vi "Wait for Stop Notification.vi"(8 "error in (no error)":errorcluster, 9 "Loop Period [ms]":i32, 11 "Event Registration Refnum in":refnum<event-registration>) -> (0 "error out":errorcluster, 1 "Stop Received?":bool, 3 "Event Registration Refnum out":refnum<event-registration>)   [LabVIEW 2020, in "Helper Loop.lvclass"]
uses:
  Helper Loop.lvclass
  Process/Protected/Broadcasting/Broadcast Message Cluster.ctl
  Broadcast Event Helpers/Broadcast Event Helpers.lvlib
  Process/Process.lvclass
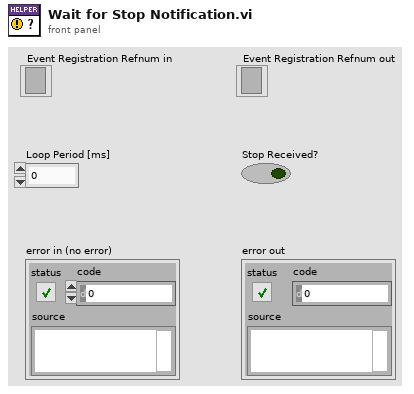
[diagram p1: front panel]
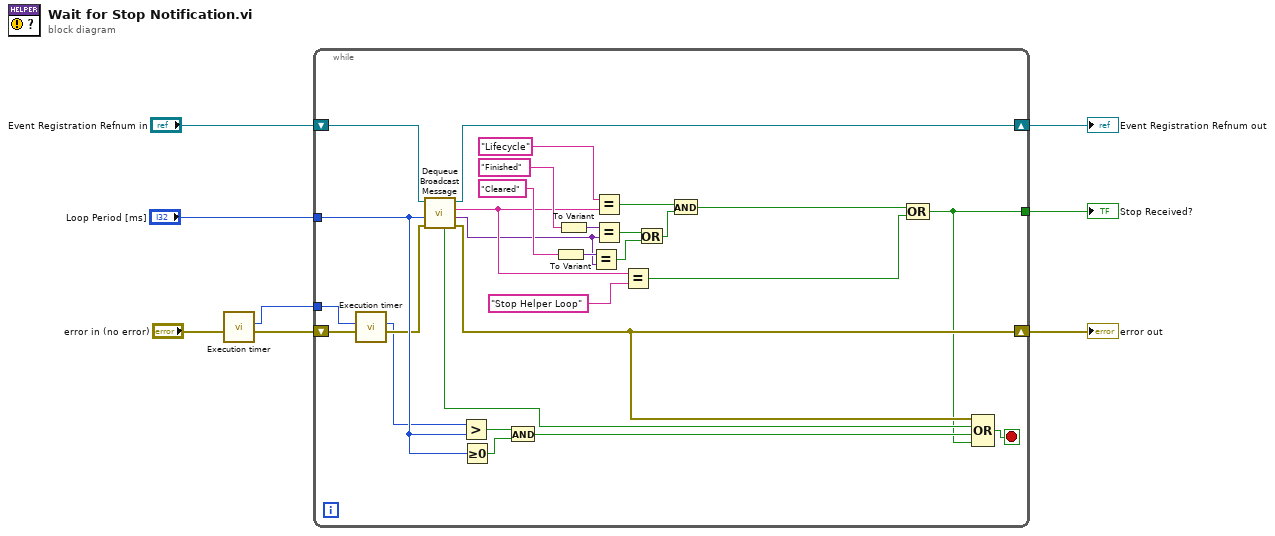
[diagram p0: block diagram]
diagram:
  n1 = call "Execution timer.vi"("error in (no error)"="error in (no error)") -> ("error out"=w1:errorcluster, "Current or Duration [ms]"=w2:u32)  [unwired: 9 in]
  n2 = while {
    tunnel: [w18] -> w8
    tunnel: "Loop Period [ms]" -> [w30]
    shift-right: [w35] -> w4
    shift-left: "Event Registration Refnum in" -> [w36]
    shift-right: [w26] -> w3
    shift-left: w1 -> [w34]
    tunnel: w2 -> [w28]
    stop <- w33 stop-if-true
    n3 = call "Execution timer.vi"("error in (no error)"=w34, "millisecond timer value"=w28) -> ("error out"=w29:errorcluster, "Current or Duration [ms]"=w27:u32)  [unwired: 8 in]
    n4 = call "Dequeue Broadcast Message.vi"("error in (no error)"=w29, "Timeout (-1)"=w30, "Event Registration Refnum"=w36) -> ("error out"=w26:errorcluster, "Message Data"=w9:variant, "Message"=w11:string, "Event Registration Refnum Out"=w35:refnum<event-registration>, "Timed Out?"=w20:bool)  [unwired: 3 in, 1 out]
    n5 = Greater?(x=w27, y=w30) -> (0:w32:bool)
    n6 = Greater Or Equal To 0?(x=w30) -> (x >= 0?=w31:bool)
    n7 = And(x=w32, y=w31) -> (x .and. y?=w19:bool)
    n8 = To Variant(anything="Cleared" ("Message")) -> (Variant=w15:variant)
    n9 = To Variant(anything="Finished" ("Message")) -> (Variant=w22:variant)
    n10 = Equal?(x=w15, y=w9) -> (x = y?=w13:bool)
    n11 = Equal?(x="Lifecycle" ("Message"), y=w11) -> (x = y?=w25:bool)
    n12 = Equal?(x=w22, y=w9) -> (x = y?=w24:bool)
    n13 = Equal?(x=w11, y="Stop Helper Loop") -> (x = y?=w21:bool)
    n14 = Or(x=w24, y=w13) -> (x .or. y?=w14:bool)
    n15 = And(x=w25, y=w14) -> (x .and. y?=w16:bool)
    n16 = Compound Arithmetic op=OR(w16, w21) -> (w18:bool)
    n17 = Compound Arithmetic op=OR(w26, w20, w19, w18) -> (w33:bool)
  }
  "Stop Received?" <- w8
  "error out" <- w3
  "Event Registration Refnum out" <- w4
